vi "Inverse Kinematics with DH_R.vi"(4 "Initial guess":dbl[](array[numeric])=[-1.0, -1.0, -1.0, -1.0], 6 "Joint Limits":dbl[][](array[numeric])=[[-68.0, -4.0], [-26.0, 52.0], [-40.0, 23.0], [-180.0, 180.0]] format="%#.3g", 7 "armID":i32, 10 "x angle(degree)":dbl, 11 "toolInsertionOffset":dbl=-54.76) -> (0 "j4":dbl, 1 "j3":dbl, 2 "j2":dbl, 3 "j1":dbl)   [LabVIEW 2016]
uses:
  RobotKinematicsDLL.dll
panel:
  out "R":dbl[][](array[numeric])=[[-1.0, -1.0, -1.0, -1.0]]
  out "pxyz":dbl[](array[numeric])=[-1.0, -1.0, -1.0, -1.0]
  out "return type":i32
  out "appended array":dbl[](array[numeric])
  out "error IO":errorcluster
  out "KINEMATICS_RET_SOLUTION_BEYOND_LIMIT":bool
  out "KINEMATICS_RET_NO_SOLUTION":bool
  out "KINEMATICS_RET_WRONG_ARM_ID":bool
  in  "x":dbl
  in  "y":dbl
  in  "z":dbl
  # ">>"
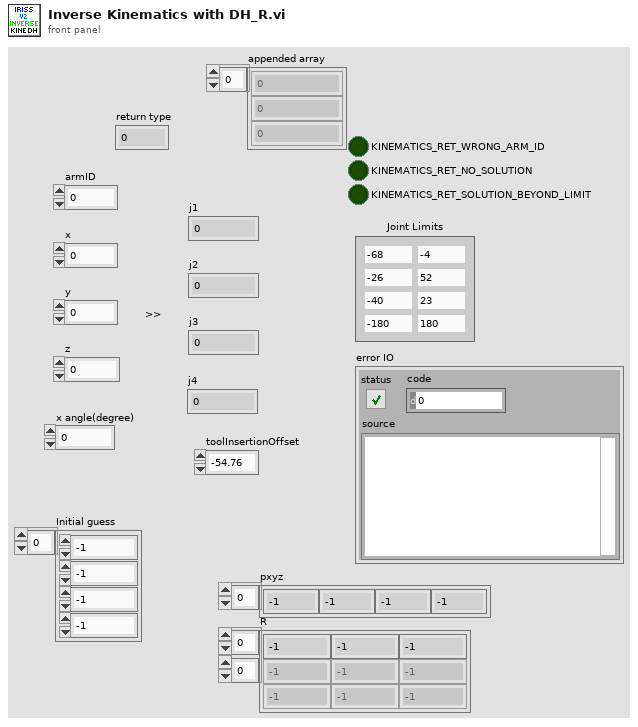
[diagram p1: front panel]
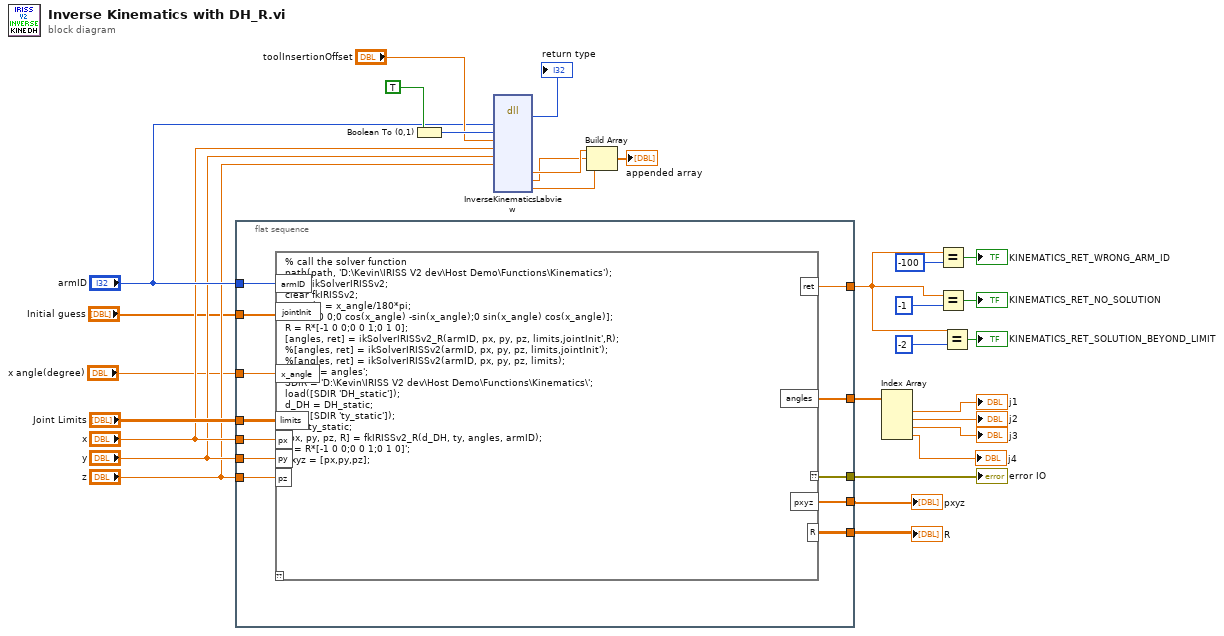
[diagram p0: block diagram]
diagram:
  n1 = flat-sequence {
    tunnel: [w39] -> w30
    tunnel: "y" -> [w42]
    tunnel: "x" -> [w41]
    tunnel: "z" -> [w40]
    tunnel: "armID" -> [w36]
    tunnel: [w38] -> w26
    tunnel: [w37] -> w18
    tunnel: "Joint Limits" -> [w35]
    tunnel: "Initial guess" -> [w34]
    tunnel: "x angle(degree)" -> [w33]
    tunnel: [w32] -> w2
    tunnel: [w31] -> w1
    frame #0 {
      n2 = script code="% call the solver function\npath(path, 'D:\\Kevin\\IRISS V2 dev\\Host Demo\\Functions\\Kinematics');\nclear ikSolverIRISSv2;\nclear fkIRISSv2;\nx_angle = x_angle/180*pi;\nR = [1 0 0;0 cos(x_angle) -sin(x_angle);0 sin(x_angle) cos(x_angle)];\nR = R*[-1 0 0;0 0 1;0 1 0];\n[angles, ret] = ikSolverIRISSv2_R(armID, px, py, pz, limits,jointInit',R);\n%[angles, ret] = ikSolverIRISSv2(armID, px, py, pz, limits,jointInit');\n%[angles, ret] = ikSolverIRISSv2(armID, px, py, pz, limits);\nangles = angles';\nSDIR = 'D:\\Kevin\\IRISS V2 dev\\Host Demo\\Functions\\Kinematics\\';\nload([SDIR 'DH_static']);\nd_DH = DH_static;\nload([SDIR 'ty_static']);\nty = ty_static;\n[px, py, pz, R] = fkIRISSv2_R(d_DH, ty, angles, armID);\nR = R*[-1 0 0;0 0 1;0 1 0]';\npxyz = [px,py,pz];"("px"=w41, "py"=w42, "pz"=w40, "armID"=w36, "limits"=w35, "jointInit"=w34, "x_angle"=w33) -> ("??"=w38:errorcluster, "angles"=w39:dbl[], "ret"=w37:dbl, "pxyz"=w32:dbl[], "R"=w31:dbl[][])  [unwired: 1 in]
    }
  }
  n3 = Boolean To (0,1)(Boolean=TRUE) -> (0, 1=w17:i16)
  n4 = dll-call lib="D:/Kevin/IRISS V2 dev/Host Demo/Functions/RobotKinematicsDLL.dll" fn="InverseKinematicsLabview"("id"="armID", "isToolInsideEye"=w17, "toolInsertionOffset"="toolInsertionOffset", "x"="x", "y"="y", "z"="z") -> ("return type"=→"return type":i32, "j1"=w8:dbl, "j2"=w7:dbl, "j3"=w6:dbl)  [unwired: 12 in, 2 out]
  n5 = Build Array(w8, w7, w6) -> (→"appended array":dbl[])
  n6 = Index Array(array=w30) -> (element #1=→"j1":dbl, element #2=→"j2":dbl, element #3=→"j3":dbl, element #4=→"j4":dbl)  [unwired: 4 in]
  n7 = Equal?(x=w18, y=-100) -> (x = y?=→"KINEMATICS_RET_WRONG_ARM_ID":bool)
  n8 = Equal?(x=w18, y=-1) -> (x = y?=→"KINEMATICS_RET_NO_SOLUTION":bool)
  n9 = Equal?(x=w18, y=-2) -> (x = y?=→"KINEMATICS_RET_SOLUTION_BEYOND_LIMIT":bool)
  "error IO" <- w26
  "pxyz" <- w2
  "R" <- w1
